vi "Counter (U32).vi"(7 "reset":bool, 9 "increment":bool=TRUE, 11 "bound":u32) -> (1 "done":bool, 3 "count out":u32)   [LabVIEW 2016]
doc: "Counts Up from 0 to <b>bound</b>."
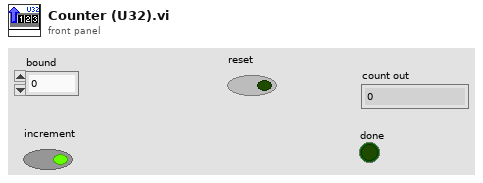
[diagram p1: front panel]
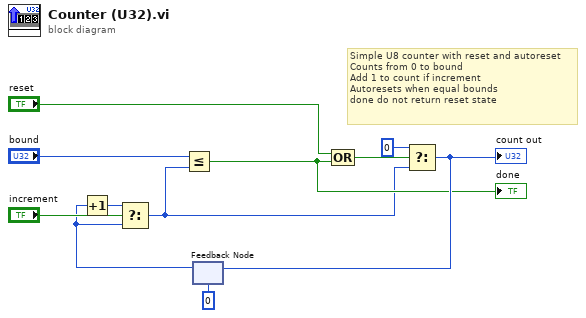
[diagram p0: block diagram]
diagram:
  # "Simple U8 counter with reset and autoreset\nCounts from 0 to bound  \nAdd 1 to count if increment\nAutoresets when equal bounds\ndone do not return reset state"
  n1 = feedback #1(u32 0 ("count in")) -> (w2:u32)
  n2 = Increment(x=w2) -> (x+1=w9:u32)
  n3 = Select(t=w9, s="increment", f=w2) -> (s? t:f=w1:u32)
  n4 = Less Or Equal?(x="bound", y=w1) -> (x <= y?=w5:bool)
  "done" <- w5
  n5 = Compound Arithmetic op=OR("reset", w5) -> (w4:bool)
  n6 = Select(t=u32 0 ("count in"), s=w4, f=w1) -> (s? t:f=w8:u32)
  "count out" <- w8
  n7 = feedback-in #1(w8) -> ()
